vi "ex_WriteDataTDMS.vi"(0 "file path":path, 1 "first call":bool, 2 "Lock file":bool=TRUE, 3 "Signals":waveform(dbl)[](array[waveform]), 4 "overwrite_mode_multi":T8(ring)=enum."overwrite & backup", 5 "overwrite_mode":T9(ring)=enum."overwrite & backup", 7 "error in (no error)":errorcluster, 8 "file dialog?":bool, 9 "Description":string, 12 "multi_file":bool, 13 "Comment":string, 14 "new file?":bool, 15 "Simulate Non-First Call":bool, 16 "file params":T6={"delimiter"="\t", "origin time"=timestamp(0 s since 1904-01-01), "Flags"={"include col headings?"=TRUE, "x_columns"=0, "col headings always?"=TRUE, "time preference"=0, "hide col headings"=FALSE}, "Decimal Separator"=""} {"Flags"."time preference" items=["Absolute", "Relative"]; "Flags"."x_columns" items=["None", "One", "Multiple"]; "origin time" format="%<%X\n%x>T"}, 23 "append info in":T5, 25 "DAQmx Task":T1) -> (17 "operator cancelled?":bool, 20 "file path out":path, 21 "bytes written":i32, 24 "append info out":T5, 27 "error out":errorcluster)   [LabVIEW 2020]
uses:
  express output/ExFileWriteBlock.llb/ex_WriteFileParams.ctl
  express input/ExFileReadBlock.llb/ex_ReadFileParams.ctl
  Platform/express/TDMExpress.llb/ex_appendInfoTDM.ctl
  ex_EditUserDefinedProperties/ex_userdefproperties.ctl
  ExFile.llb/ex_userDefProperty.ctl
  ex_EditUserDefinedProperties/usiDataType.ctl
  ExFile.llb/ex_propertySource.ctl
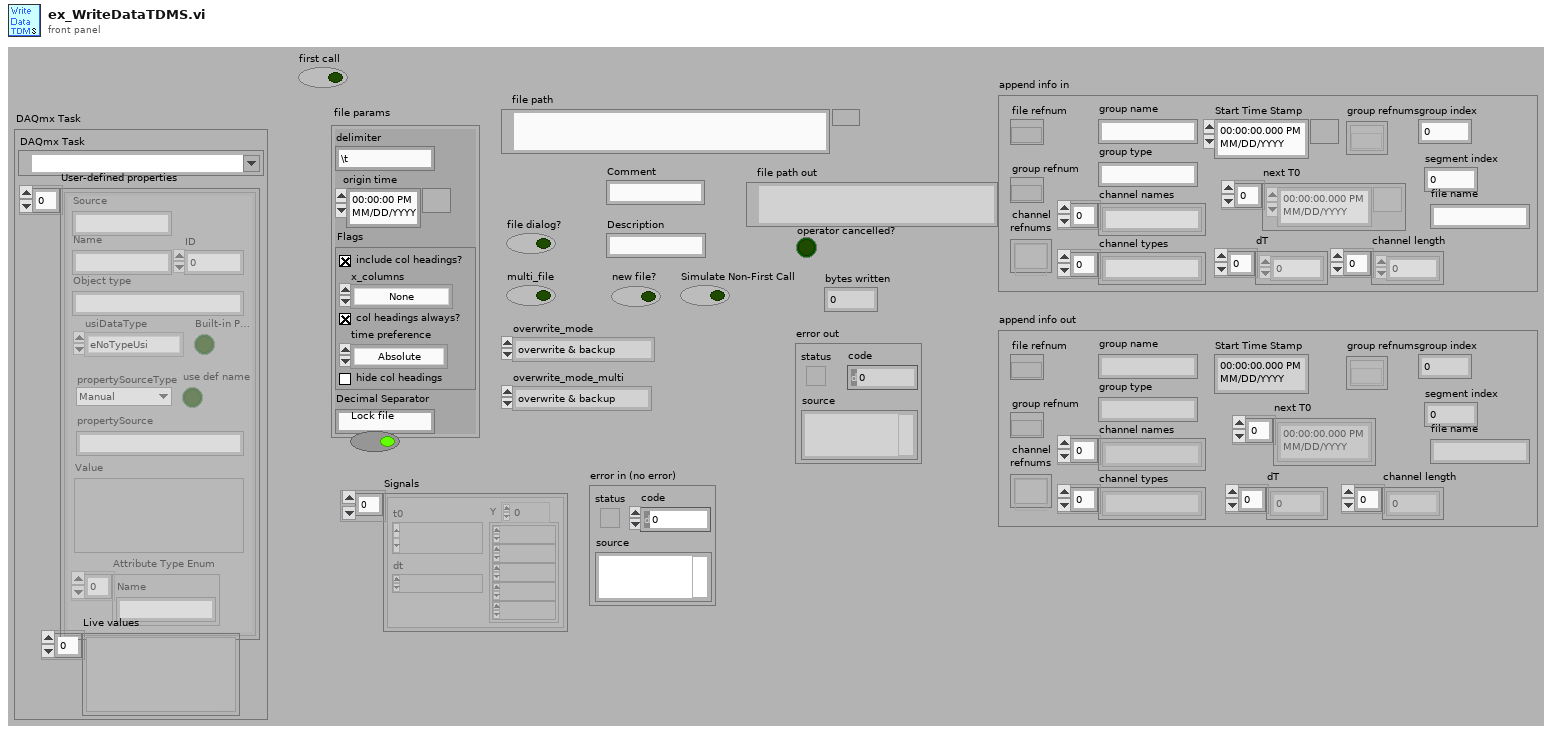
[diagram p1: front panel]
types:
  T1 = typedef "ex_userdefproperties.ctl" = cluster{"DAQmx Task":refnum<k21>, "User-defined properties":T2[], "Live values":variant[]}
  T2 = typedef "ex_userDefProperty.ctl" = cluster{"Name":string, "Object type":string, "usiDataType":T3, "propertySourceType":T4, "propertySource":string, "Value":variant, "ID":i32, "use def name":bool, "Source":string, "Built-in Prop":bool, "Attribute Type Enum":string[]}
  T3 = typedef "usiDataType.ctl" = enum16{"eNoTypeUsi", "eInt8Usi", "eInt16Usi", "eInt32Usi", "eInt64Usi", "eUInt8Usi", "eUInt16Usi", "eUInt32Usi", "eUInt64Usi", "eFloat32Usi", "eFloat64Usi", "- 0", "- 1", "- 2", "- 3", "- 4", "- 5", "- 6", "- 7", "- 8", "- 9", "eString8Usi", "eString16Usi", "eStringUsi", "eEnumUsi", "- 10", "- 11", "- 12", "- 13", "- 14", "eTimeUsi", "- 15", "- 16", "- 17", "- 18", "- 19", "- 20", "- 21", "- 22", "- 23", "eInstanceUsi", "eStoreUsi"}
  T4 = typedef "ex_propertySource.ctl" = enum16{"Manual", "System", "DAQmx Channel", "Terminal", "Ignore"}
  T5 = typedef "ex_appendInfoTDM.ctl" = cluster{"channel\nrefnums":refnum<k20>[], "channel names":string[], "channel types":string[], "file refnum":refnum<k20>, "group refnum":refnum<k20>, "group name":string, "group type":string, "next T0":timestamp[], "dT":dbl[], "Start Time Stamp":timestamp, "channel length":u32[], "group index":u32, "group refnums":refnum<k20>[], "file name":string, "segment index":u32}
  T6 = typedef "ex_WriteFileParams.ctl" = cluster{"delimiter":string, "origin time":timestamp, "Flags":T7, "Decimal Separator":string}
  T7 = typedef "ex_ReadFileParams.ctl" = cluster{"include col headings?":bool, "x_columns":u16, "col headings always?":bool, "time preference":u16, "hide col headings":bool}
  T8 = enum16{"overwrite", "overwrite & backup", "next avail"}
  T9 = enum16{"overwrite", "overwrite & backup", "append", "next avail"}
  T10 = cluster{"Start Timestamp":timestamp, "Timestamp":timestamp, "Relative Time?":bool, "X Dimension":string, "Signal Name":string, "Y Units":string, "X0":timestamp, "dX":dbl, "nPoints":i32}[]
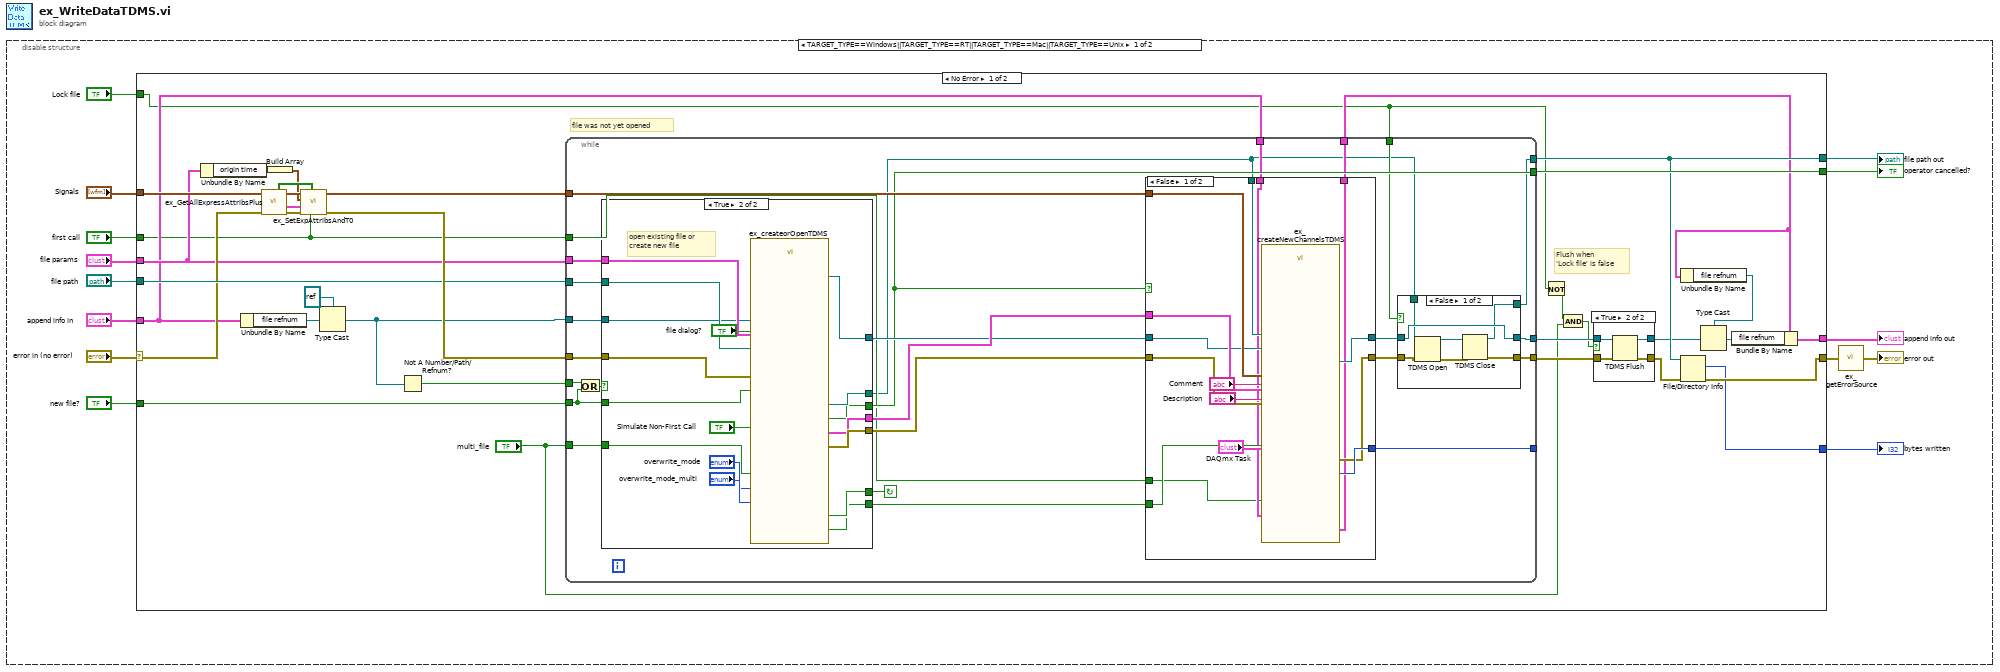
[diagram p0: block diagram]
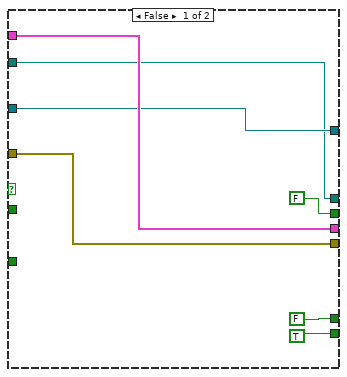
[diagram p3: hidden frame]
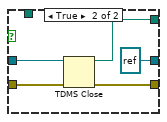
[diagram p4: hidden frame]
diagram:
  n1 = disable-structure shown="TARGET_TYPE==Windows||TARGET_TYPE==RT||TARGET_TYPE==Mac||TARGET_TYPE==Unix" {
    frame condition #0 (active) {
      n2 = case shown="No Error" "error in (no error)" {
        selector: "error in (no error)" -> [w38 w138]
        tunnel: [w27 w138] -> w14
        tunnel: "Signals" -> [w40 _]
        tunnel: "new file?" -> [w47 _]
        tunnel: "file params" -> [w32 _]
        tunnel: [w31 w137] -> w7
        tunnel: "file path" -> [w48 w136]
        tunnel: "append info in" -> [w29 w137]
        tunnel: "Lock file" -> [w16 _]
        tunnel: [w26 w136] -> w6
        tunnel: [w45 _] -> w5
        tunnel: [w25 _] -> w4
        tunnel: "first call" -> [w28 _]
        frame No Error {
          # "Flush when \n'Lock file' is false"
          # "file was not yet opened"
          n3 = Unbundle By Name(w32) -> ("origin time"=w37:timestamp)
          n4 = Unbundle By Name(w29) -> ("file refnum"=w35:refnum<k20>)
          n5 = call "ex_GetAllExpressAttribsPlus.vi"("error in"=w38, "Signals in"=w40) -> ("error out"=w44:errorcluster, "All Express Wave Attributes Plus"=w43:T10, "Signals out"=w42:waveform(dbl)[], "Time Attribs Not Found"=w41:bool[])  [unwired: 6 out]
          n6 = Build Array(w37) -> (w36:timestamp[])
          n7 = call "ex_SetExpAttribsAndT0.vi"("Latch Origin TS? (T)"=w28, "Set? (T if empty)"=w41, "error in (no error)"=w44, "Express Attributes Plus in"=w43, "Origin Timestamps"=w36, "Signals"=w42) -> ("error out"=w49:errorcluster, "Signals With Attributes"=w39:waveform(dbl)[])  [unwired: 4 out]
          n8 = Type Cast(type=refnum<k34> refnum ("tdms file out"), x=w35) -> (*(type *) &x=w33:refnum<k34>)
          n9 = Not A Number/Path/Refnum?(number/path/refnum=w33) -> (NaN/Path/Refnum?=w46:bool)
          n10 = while {
            tunnel: w49 -> [w81]
            tunnel: w47 -> [w67]
            tunnel: w48 -> [w80]
            tunnel: [w58] -> w26
            tunnel: [w63] -> w45
            tunnel: [w76] -> w20
            tunnel: [w79] -> _
            tunnel: w32 -> [w78]
            tunnel: [w75] -> w22
            tunnel: w16 -> [w59]
            tunnel: w33 -> [w71]
            tunnel: w39 -> [w72]
            tunnel: w46 -> [w68]
            tunnel: w29 -> [w62]
            tunnel: [w61] -> w24
            tunnel: w28 -> [w60]
            tunnel: "multi_file" -> [w56]
            stop <- w77 continue-if-true
            n11 = Or(x=w68, y=w67) -> (x .or. y?=w69:bool)
            n12 = case shown="True" w69 {
              tunnel: w81 -> [w86 w105]
              tunnel: w80 -> [w85 w104]
              tunnel: w78 -> [w88 w102]
              tunnel: [FALSE ("keep loop going") w98] -> w77
              tunnel: [w85 w97] -> w57
              tunnel: [w86 w96] -> w74
              tunnel: [w88 w95] -> w73
              tunnel: w67 -> [_ w94]
              tunnel: w71 -> [w87 w93]
              tunnel: [w87 w92] -> w70
              tunnel: [FALSE ("dialog was cancelled") w91] -> w63
              tunnel: [TRUE ("keep loop going") w90] -> w66
              tunnel: w56 -> [_ w89]
              frame False {
              }
              frame True {
                # "open existing file or\ncreate new file"
                n13 = call "ex_createorOpenTDMS.vi"("file path in"=w104, "overwrite_mode_multi"="overwrite_mode_multi", "overwrite_mode"="overwrite_mode", "tdms file in"=w93, "file dialog?"="file dialog?", "error in (no error)"=w105, "file params"=w102, "multi_file"=w89, "new file?"=w94, "Simulate Non-First Call"="Simulate Non-First Call") -> ("new file was created"=w90:bool, "file path out"=w97:path, "dialog was cancelled"=w91:bool, "keep loop going"=w98:bool, "tdms file out"=w92:refnum<k34>, "file params out"=w95:T6, "error out"=w96:errorcluster)  [unwired: 3 out]
              }
            }
            n14 = case shown="False" w63 {
              tunnel: w73 -> [w128 _]
              tunnel: [w130 w135] -> w64
              tunnel: w74 -> [w132 w135]
              tunnel: [w131 _] -> w79
              tunnel: [w129 w134] -> w65
              tunnel: w70 -> [w121 w134]
              tunnel: w72 -> [w127 _]
              tunnel: w66 -> [w126 _]
              tunnel: w57 -> [w122 _]
              tunnel: w62 -> [w120 w133]
              tunnel: [w119 w133] -> w61
              tunnel: w60 -> [w118 _]
              frame False {
                n15 = call "ex_createNewChannelsTDMS.vi"("DAQmx Task"="DAQmx Task", "tdms file in"=w121, "append info in"=w120, "signals"=w127, "file params"=w128, "File path"=w122, "is first call"=w118, "error in (no error)"=w132, "Comment"="Comment", "Description"="Description", "write file properties"=w126) -> ("append info out"=w119:T5, "tdms file out"=w129:refnum<k34>, "bytes written"=w131:i32, "error out"=w130:errorcluster)  [unwired: 1 out]
              }
              frame True {
              }
            }
            n16 = case shown="False" w59 {
              tunnel: w64 -> [w111 w117]
              tunnel: [w109 w115] -> w76
              tunnel: w65 -> [w112 w116]
              tunnel: [w112 refnum<k34> refnum ("tdms file out")] -> w75
              tunnel: [w107 w113] -> w58
              tunnel: w57 -> [w106 _]
              frame False {
                n17 = TDMS Open(8:w111, 11:w106) -> (0:w110:errorcluster, 3:w108:refnum<k34>)  [unwired: 5 in]
                n18 = TDMS Close(8:w110, 11:w108) -> (0:w109:errorcluster, 3:w107:path)
              }
              frame True {
                n19 = TDMS Close(8:w117, 11:w116) -> (0:w115:errorcluster, 3:w113:path)
              }
            }
          }
          n20 = Not(x=w16) -> (.not. x?=w15:bool)
          n21 = And(x=w15, y="multi_file") -> (x .and. y?=w17:bool)
          n22 = case shown="True" w17 {
            tunnel: w22 -> [w51 w55]
            tunnel: [w51 w54] -> w21
            tunnel: w20 -> [w50 w53]
            tunnel: [w50 w52] -> w19
            frame False {
            }
            frame True {
              n23 = TDMS Flush(4:w53, 7:w55) -> (0:w52:errorcluster, 3:w54:refnum<k34>)
            }
          }
          n24 = Unbundle By Name(w24) -> ("file refnum"=w23:refnum<k20>)
          n25 = File/Directory Info(path=w26, error in=w19) -> (size=w25:i64, error out=w27:errorcluster)  [unwired: 5 out]
          n26 = Type Cast(type=w23, x=w21) -> (*(type *) &x=w30:refnum<k20>)
          n27 = Bundle By Name(cluster=w24, "file refnum"=w30) -> (w31:T5)
        }
        frame Error {
        }
      }
      "append info out" <- w7
      "operator cancelled?" <- w5
      "file path out" <- w6
      "bytes written" <- w4
      n28 = call "ex_getErrorSource.vi"("error in (no error)"=w14) -> ("error out"=→"error out":errorcluster)
    }
    frame condition #1 {
    }
  }
